vi "SetFilepath.vi"(10 "Array 2":string[](array[string]), 11 "Array":refnum<vi>[](array[refnum])) -> ()   [LabVIEW 2017]
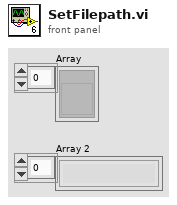
[diagram p1: front panel]
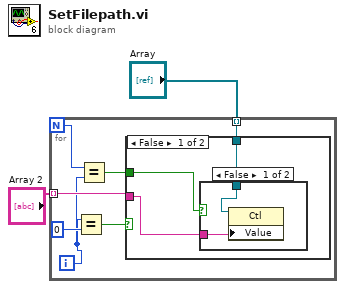
[diagram p0: block diagram]
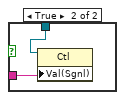
[diagram p2: hidden frame]
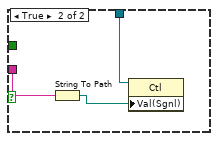
[diagram p3: hidden frame]
diagram:
  n1 = for {
    N -> [w5]
    tunnel: "Array 2" -> [w7] mode=indexing
    tunnel: "Array" -> [w6] mode=indexing
    i -> [w3]
    n2 = Equal?(x=w3, y=0) -> (x = y?=w9:bool)
    n3 = Equal?(x=w5, y=w3) -> (x = y?=w4:bool)
    n4 = case shown="False" w9 {
      tunnel: w7 -> [w11 w19]
      tunnel: w6 -> [w12 w18]
      tunnel: w4 -> [w10 _]
      frame False {
        n5 = case shown="False" w10 {
          tunnel: w12 -> [w14 w16]
          tunnel: w11 -> [w13 w15]
          frame False {
            n6 = property class="Ctl"(reference=w14, "Value"=w13) -> ()  [unwired: 1 in, 2 out]
          }
          frame True {
            n7 = property class="Ctl"(reference=w16, "Val(Sgnl)"=w15) -> ()  [unwired: 1 in, 2 out]
          }
        }
      }
      frame True {
        n8 = String To Path(string=w19) -> (path=w17:path)
        n9 = property class="Ctl"(reference=w18, "Val(Sgnl)"=w17) -> ()  [unwired: 1 in, 2 out]
      }
    }
  }
